vi "Freefield-Show all.vi"(0 "Path":path, 5 "Mag graph":refnum<vi>, 7 "Phase graph":refnum<vi>, 11 "error in (no error)":errorcluster) -> (15 "error out":errorcluster)   [LabVIEW 2020]
doc: "This helper VI plots all of the in ear calibration files in the current experiment data folder.\n\nKEH 9/10/09"
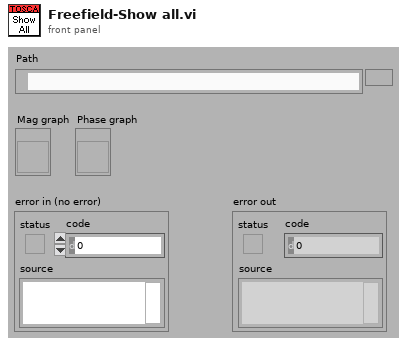
[diagram p1: front panel]
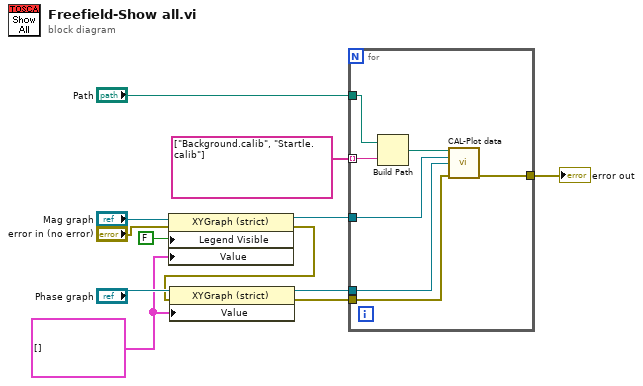
[diagram p0: block diagram]
diagram:
  w8 = cluster{"PTC Mag":dbl[], "PTC Phase":dbl[]}[] [] ("Value")
  n1 = property class="XYGraph (strict)"(reference="Mag graph", error in="error in (no error)", "Legend Visible"=FALSE ("Legend:Visible"), "Value"=w8) -> (reference out=w4:refnum<vi>, error out=w7:errorcluster)
  n2 = property class="XYGraph (strict)"(reference="Phase graph", error in=w7, "Value"=w8) -> (reference out=w3:refnum<vi>, error out=w2:errorcluster)
  n3 = for {
    tunnel: string[] ["Background.calib", "Startle.calib"] -> [w18] mode=indexing
    tunnel: "Path" -> [w19]
    tunnel: w4 -> [w16]
    tunnel: w3 -> [w15]
    tunnel: w2 -> [w14]
    tunnel: [w13] -> w1
    n4 = Build Path(base path=w19, name or relative path=w18) -> (appended path=w17:path)
    n5 = call "CAL-Plot data.vi"("Path"=w17, "Mag graph"=w16, "Phase graph"=w15, "error in (no error)"=w14) -> ("error out"=w13:errorcluster)  [unwired: 10 in, 1 out]
  }
  "error out" <- w1
